vi "Versioned Write.vi"(9 "MEGA Path Stuff":T10(array[cluster]) {"?"."Limits"."StoopidFast (fps)" min=0.0; "?"."Limits"."Jerk (fps^3)" min=0.0 step=1.0; "?"."Limits"."Accel (fps^2)" min=0.0; "?"."Limits"."Velocity (fps)" min=0.0; "?"."Overrides"."Angle Override" step=5.0; "?"."Overrides"."Velocity Override" step=5.0; "?"."Overrides"."Angular Override" step=5.0; "?"."Angular Limits"."Jerk (deg/s^3)" min=0.0 step=1.0; "?"."Angular Limits"."Accel (deg/s^2)" min=0.0; "?"."Angular Limits"."Velocity (deg/s)" min=0.0}, 10 "Filename":string, 11 "Bordeaux paths in":path) -> ()   [LabVIEW 2023]
uses:
  Types/Trajectory Data.ctl
  Types/Segment Type.ctl
  Types/Single Cmd Info.ctl
  <vilib>/picture/picture.llb/imagedata.ctl
  Types/Limits.ctl
  Types/Overrides.ctl
  Types/Angluar Limits.ctl
  Types/Drive Type.ctl
  Types/Path Type.ctl
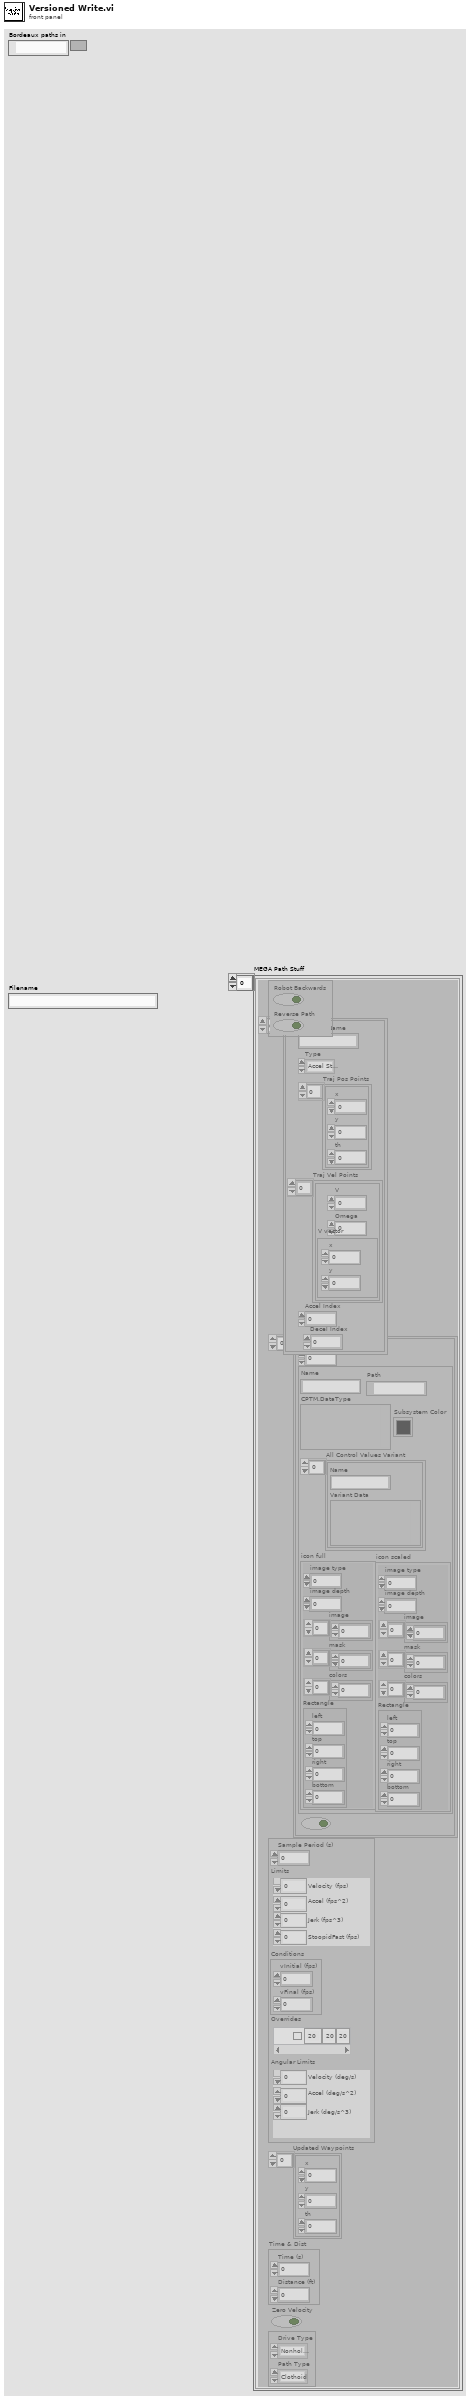
[diagram p1: front panel]
types:
  T1 = typedef "Trajectory Data.ctl" = cluster{"Segment Name":string, "Type":T2, "Traj Pos Points":cluster{"x":dbl, "y":dbl, "th":dbl}[], "Traj Vel Points":cluster{"V":dbl, "Omega":dbl, "V vector":cluster{"y":dbl, "x":dbl}}[], "Accel Index":i32, "Decel Index":i32}[]
  T2 = typedef "Segment Type.ctl" = enum16{"Accel Straight", "Const Straight", "Blend", "Circle", "Bezier"}
  T3 = typedef "Single Cmd Info.ctl" = cluster{"Name":string, "CPTM.DataType":variant, "All Control Values Variant":cluster{"Name":string, "Variant Data":variant}[], "icon full":T4, "icon scaled":T4, "Path":path, "Subsystem Color":u32}
  T4 = typedef "imagedata.ctl" = cluster{"image type":i32, "image depth":i32, "image":u8[], "mask":u8[], "colors":u32[], "Rectangle":cluster{"left":i16, "top":i16, "right":i16, "bottom":i16}}
  T5 = typedef "Limits.ctl" = cluster{"Velocity (fps)":dbl, "Accel (fps^2)":dbl, "Jerk (fps^3)":dbl, "StoopidFast (fps)":dbl}
  T6 = typedef "Overrides.ctl" = cluster{"Count":string, "Angular Override":dbl, "Enabled?":bool, "Velocity Override":dbl, "Angle Override":dbl}[]
  T7 = typedef "Angluar Limits.ctl" = cluster{"Velocity (deg/s)":dbl, "Accel (deg/s^2)":dbl, "Jerk (deg/s^3)":dbl}
  T8 = typedef "Drive Type.ctl" = enum16{"Nonholonomic", "Holonomic"}
  T9 = typedef "Path Type.ctl" = enum16{"Clothoid", "Bezier"}
  T10 = cluster{cluster{"Robot Backwards":bool, "Reverse Path":bool}, "Trajectory Data":T1, "Commands out":cluster{"Time (s)":dbl, T3, bool}[], cluster{"Sample Period (s)":dbl, "Limits":T5, "Conditions":cluster{"vInitial (fps)":dbl, "vFinal (fps)":dbl}, "Overrides":T6, "Angular Limits":T7}, "Updated Waypoints":cluster{"x":dbl, "y":dbl, "th":dbl}[], "Time & Dist":cluster{"Time (s)":dbl, "Distance (ft)":dbl}, "Zero Velocity":bool, cluster{"Drive Type":T8, "Path Type":T9}}[]
  T11 = cluster{"Robot Backwards":bool, "Reverse Path":bool}
  T12 = cluster{"Sample Period (s)":dbl, "Limits":T5, "Conditions":cluster{"vInitial (fps)":dbl, "vFinal (fps)":dbl}, "Overrides":T6, "Angular Limits":T7}
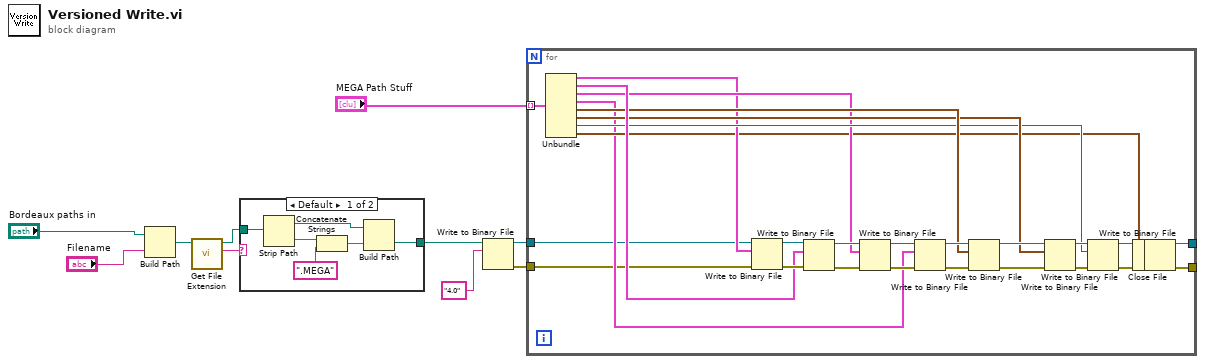
[diagram p0: block diagram]
diagram:
  n1 = Build Path(base path="Bordeaux paths in", name or relative path="Filename") -> (appended path=w10:path)
  n2 = call <vilib>:"Get File Extension.vi"("file"=w10) -> ("lowercase file extension"=w11:string, "dup file"=w12:path)  [unwired: 6 in, 3 out]
  n3 = case shown="Default" w11 {
    tunnel: w12 -> [w17 w19]
    tunnel: [w14 w19] -> w3
    frame Default {
      n4 = Strip Path(path=w17) -> (stripped path=w15:path, name=w16:string)
      n5 = Concatenate Strings(w16, ".MEGA") -> (w13:string)
      n6 = Build Path(base path=w15, name or relative path=w13) -> (appended path=w14:path)
    }
    frame "bdx" {
    }
  }
  n7 = Write to Binary File(file (use dialog)=w3, data="4.0") -> (refnum out=w1:refnum<file>, error out=w2:errorcluster)  [unwired: 4 in, 1 out]
  n8 = for {
    tunnel: "MEGA Path Stuff" -> [w28] mode=indexing
    tunnel: [w26] -> w6
    tunnel: [w24] -> w5
    tunnel: w2 -> [w21]
    tunnel: w1 -> [w20]
    n9 = Unbundle(w28) -> (w29:T11, "Trajectory Data"=w34:T1, "Commands out"=w30:cluster{"Time (s)":dbl, T3, bool}[], w22:T12, "Updated Waypoints"=w33:cluster{"x":dbl, "y":dbl, "th":dbl}[], "Time & Dist"=w32:cluster{"Time (s)":dbl, "Distance (ft)":dbl}, "Zero Velocity"=w31:bool, w23:cluster{"Drive Type":T8, "Path Type":T9})
    n10 = Write to Binary File(file (use dialog)=w20, data=w29, error in=w21) -> (refnum out=w37:refnum<file>, error out=w41:errorcluster)  [unwired: 3 in, 1 out]
    n11 = Write to Binary File(file (use dialog)=w37, data=w34, error in=w41) -> (refnum out=w38:refnum<file>, error out=w42:errorcluster)  [unwired: 3 in, 1 out]
    n12 = Write to Binary File(file (use dialog)=w38, data=w30, error in=w42) -> (refnum out=w39:refnum<file>, error out=w43:errorcluster)  [unwired: 3 in, 1 out]
    n13 = Write to Binary File(file (use dialog)=w39, data=w22, error in=w43) -> (refnum out=w35:refnum<file>, error out=w44:errorcluster)  [unwired: 3 in, 1 out]
    n14 = Write to Binary File(file (use dialog)=w35, data=w33, error in=w44) -> (refnum out=w36:refnum<file>, error out=w45:errorcluster)  [unwired: 3 in, 1 out]
    n15 = Write to Binary File(file (use dialog)=w36, data=w32, error in=w45) -> (refnum out=w40:refnum<file>, error out=w46:errorcluster)  [unwired: 3 in, 1 out]
    n16 = Write to Binary File(file (use dialog)=w40, data=w31, error in=w46) -> (refnum out=w27:refnum<file>, error out=w25:errorcluster)  [unwired: 3 in, 1 out]
    n17 = Write to Binary File(file (use dialog)=w27, data=w23, error in=w25) -> (refnum out=w26:refnum<file>, error out=w24:errorcluster)  [unwired: 3 in, 1 out]
  }
  n18 = Close File(refnum=w6, error in=w5) -> ()  [unwired: 2 out]
